vi "HTTPGET请求转换经纬度.vi"(10 "字符串 2":string, 11 "字符串":string) -> (3 "body":string)   [LabVIEW 2015]
uses:
  <vilib>/httpClient/LabVIEWHTTPClient.lvlib
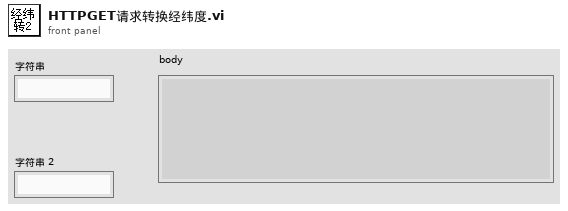
[diagram p1: front panel]
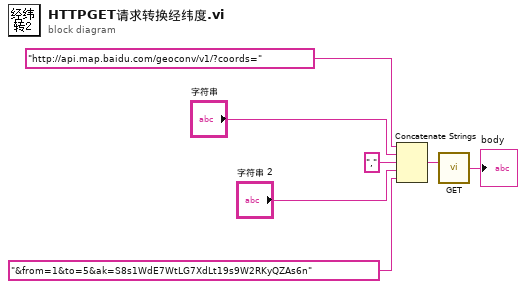
[diagram p0: block diagram]
diagram:
  n1 = Concatenate Strings("http://api.map.baidu.com/geoconv/v1/?coords=" ("url"), "字符串", "," ("url"), "字符串 2", "&from=1&to=5&ak=S8s1WdE7WtLG7XdLt19s9W2RKyQZAs6n" ("url")) -> (w1:string)
  n2 = call <vilib>:"GET.vi"("url"=w1) -> ("body"=→"body":string)  [unwired: 11 in, 3 out]
